vi "Create.vi"(8 "error in":errorcluster, 10 "Index":u16 format="%.0x") -> (0 "error out":errorcluster, 3 "Object Entry":refnum<class "Object Entry.lvclass">)   [LabVIEW 2020, in "CANopen.lvlib" / "Object Entry.lvclass"]
uses:
  Object Entry.lvclass
  Object Entry.lvclass/Object Entry.ctl
  Sub Object/Sub Object.lvclass
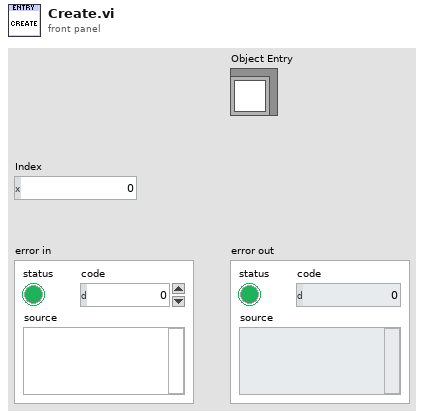
[diagram p1: front panel]
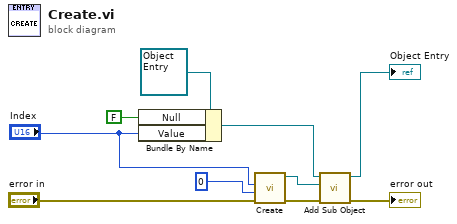
[diagram p0: block diagram]
diagram:
  n1 = Bundle By Name(cluster=refnum<class "Object Entry.lvclass"> refnum ("Object Entry"), "Null"=FALSE ("Index.Null"), "Value"="Index") -> (w5:refnum<class "Object Entry.lvclass">)
  n2 = call "Create.vi"("error in"="error in", "Sub Index"=u8 0, "Index"="Index") -> ("error out"=w7:errorcluster, "Sub Obj out"=w3:refnum<class "Sub Object.lvclass">)  [unwired: 7 in]
  n3 = call "Add Sub Object.vi"("error in"=w7, "Sub Object"=w3, "Obj Entry in"=w5) -> ("error out"=→"error out":errorcluster, "Obj Entry out"=→"Object Entry":refnum<class "Object Entry.lvclass">)  [unwired: 7 in]
